vi "dbc-check-baud-rate.vi"(8 "error in (no error)":errorcluster, 9 "XNET Cluster 2":refnum<k21>, 11 "dbc in":refnum<class "dbc.lvclass">) -> (0 "error out":errorcluster, 3 "dbc out":refnum<class "dbc.lvclass">)   [LabVIEW 2015, in "dbc.lvclass"]
uses:
  dbc.lvclass
  class.bFrameIO/bFrameIO.lvclass/bFrameIO.ctl
  class.bFrameIO/wrt-baud-rate.vi
  class.bFrameIO/read-baud-rate.vi
  class.bFrameIO/wrt-fi-cluster.vi
  <resource>/objmgr/xnet.rc
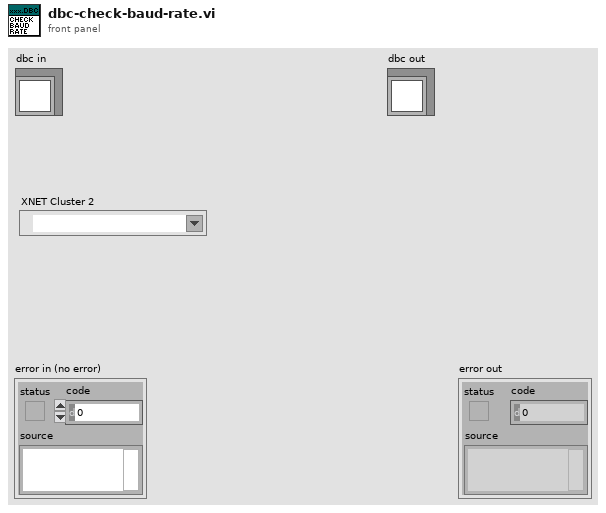
[diagram p1: front panel]
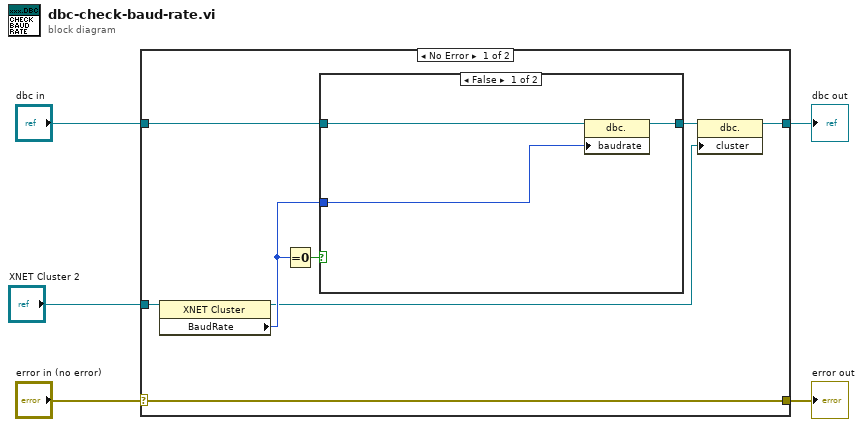
[diagram p0: block diagram]
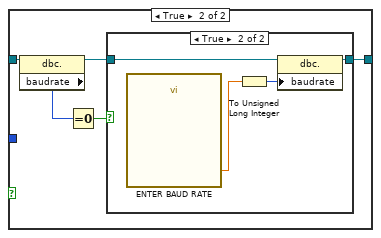
[diagram p2: hidden frame]
diagram:
  n1 = case shown="No Error" "error in (no error)" {
    selector: "error in (no error)" -> [w13 w28]
    tunnel: [w13 w28] -> w4
    tunnel: [w7 w27] -> w2
    tunnel: "dbc in" -> [w8 w27]
    tunnel: "XNET Cluster 2" -> [w12 _]
    frame No Error {
      n2 = property class="XNET Cluster"(reference=w12) -> (reference out=w6:refnum<k21>, "BaudRate"=w10:u32)  [unwired: 1 in, 1 out]
      n3 = Equal To 0?(x=w10) -> (x = 0?=w11:bool)
      n4 = case shown="False" w11 {
        tunnel: w10 -> [w14 _]
        tunnel: [w15 w20] -> w9
        tunnel: w8 -> [w16 w21]
        frame False {
          n5 = property class="dbc."(reference=w16, "baudrate"=w14) -> (reference out=w15:refnum<class "dbc.lvclass">)  [unwired: 1 in, 1 out]
        }
        frame True {
          n6 = property class="dbc."(reference=w21) -> (reference out=w19:refnum<class "dbc.lvclass">, "baudrate"=w17:u32)  [unwired: 1 in, 1 out]
          n7 = Equal To 0?(x=w17) -> (x = 0?=w18:bool)
          n8 = case shown="True" w18 {
            tunnel: w19 -> [w22 w25]
            tunnel: [w22 w24] -> w20
            frame False {
            }
            frame True {
              n9 = call "ENTER BAUD RATE"() -> ("baudrate"=w26:dbl)  [unwired: 17 in, 2 out]
              n10 = To Unsigned Long Integer(number=w26) -> (unsigned 32bit integer=w23:u32)
              n11 = property class="dbc."(reference=w25, "baudrate"=w23) -> (reference out=w24:refnum<class "dbc.lvclass">)  [unwired: 1 in, 1 out]
            }
          }
        }
      }
      n12 = property class="dbc."(reference=w9, "cluster"=w6) -> (reference out=w7:refnum<class "dbc.lvclass">)  [unwired: 1 in, 1 out]
    }
    frame Error {
    }
  }
  "error out" <- w4
  "dbc out" <- w2
